vi "sweep init checklist.vi"(9 "list":string[](array[string])=["tabs: init", "gas flow: init", "PID: init", "save log: init", "overheat: init", "counter: init", "sweep table: init", "9ctl: init"], 10 "init str":string, 11 "action":string="action") -> (3 "result":bool)   [LabVIEW 2015]
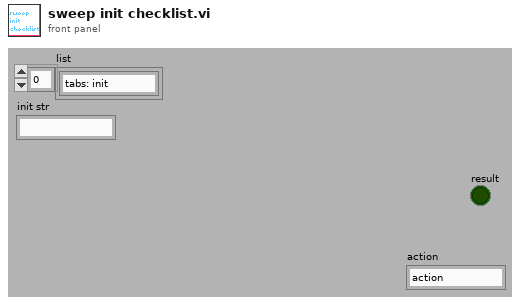
[diagram p1: front panel]
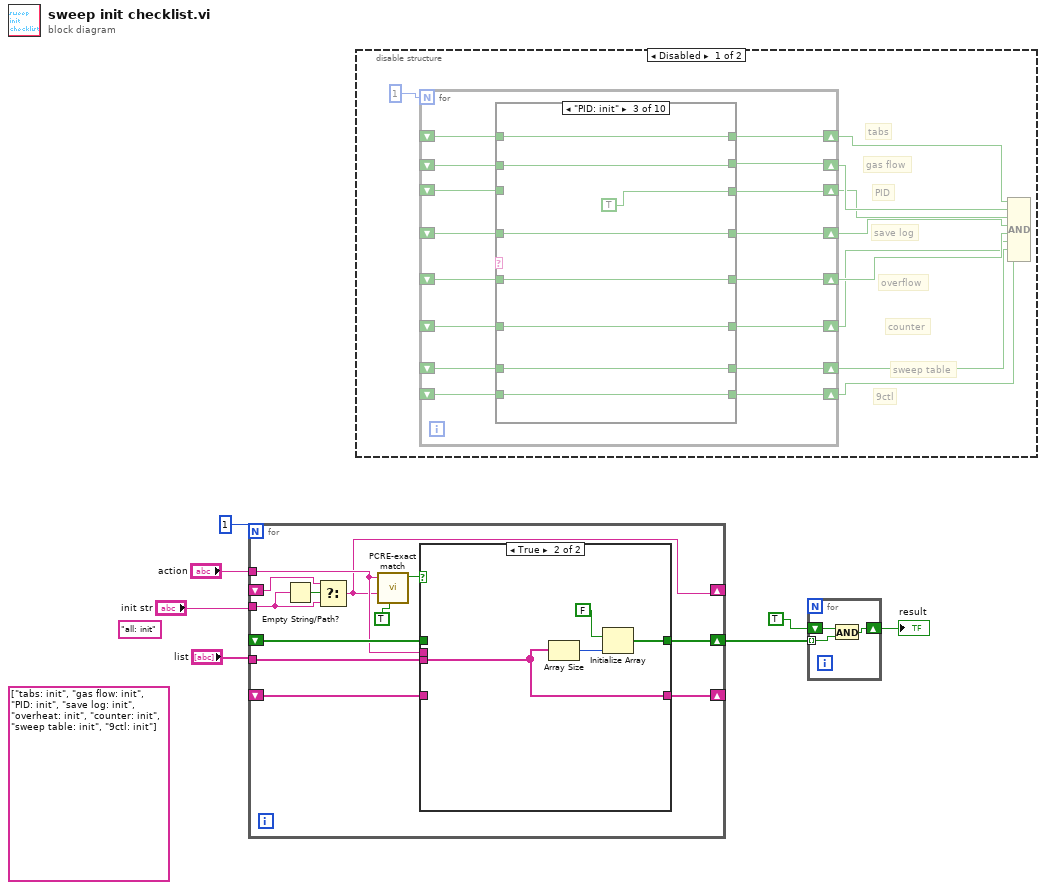
[diagram p0: block diagram]
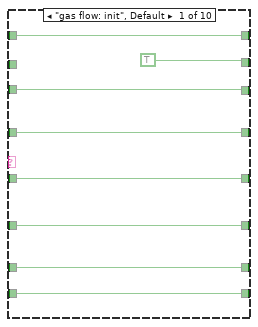
[diagram p2: hidden frame]
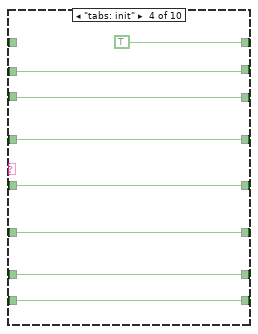
[diagram p4: hidden frame]
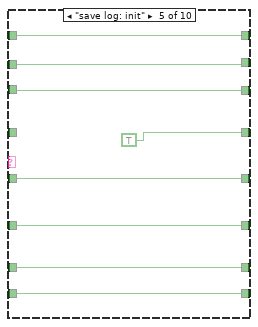
[diagram p5: hidden frame]
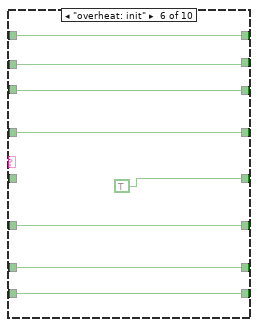
[diagram p6: hidden frame]
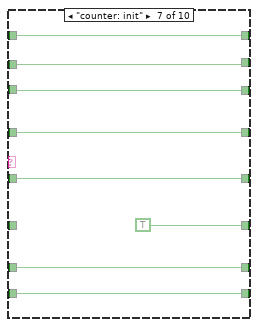
[diagram p7: hidden frame]
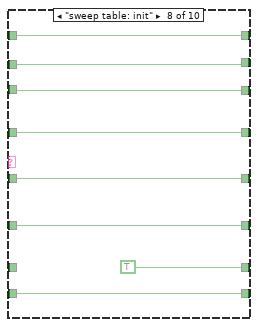
[diagram p8: hidden frame]
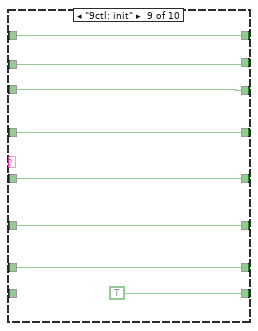
[diagram p9: hidden frame]
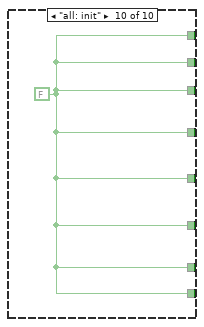
[diagram p10: hidden frame]
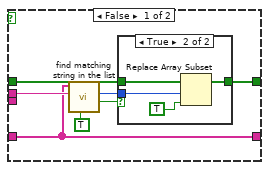
[diagram p12: hidden frame]
diagram:
  (unwired) "all: init" ("regular expression")
  (unwired) string[] ["tabs: init", "gas flow: init", "PID: init", "save log: init", "overheat: init", "counter: init", "sweep table: init", "9ctl: init"]
  n1 = for {
    N: 1 -> [_]
    tunnel: "action" -> [w12]
    shift-right: [w14] -> w5
    shift-left: _ -> [w17]
    shift-right: [w13] -> _
    shift-left: _ -> [w15]
    tunnel: "list" -> [w16]
    tunnel: "init str" -> [w9]
    shift-right: [w8] -> _
    shift-left: _ -> [w10]
    n2 = Empty String/Path?(string/path=w9) -> (empty?=w11:bool)
    n3 = Select(t=w10, s=w11, f=w9) -> (s? t:f=w8:string)
    n4 = call "PCRE-exact match.vi"("quote specials"=TRUE, "regular expression"=w8, "input string"=w12) -> ("exact match"=w18:bool)  [unwired: 6 in, 2 out]
    n5 = case shown="True" w18 {
      tunnel: [w20 w35] -> w14
      tunnel: w17 -> [w22 _]
      tunnel: [w21 w32] -> w13
      tunnel: w16 -> [_ w32]
      tunnel: w15 -> [w21 _]
      tunnel: w12 -> [w23 _]
      frame False {
        n6 = call "find matching string in the list.vi"("quote specials"=TRUE, "regular expression"=w23, "strings"=w21) -> ("match found"=w25:bool, "matching string index"=w26:i32)  [unwired: 6 in, 1 out]
        n7 = case shown="True" w25 {
          tunnel: w26 -> [_ w30]
          tunnel: [w27 w29] -> w20
          tunnel: w22 -> [w27 w28]
          frame False {
          }
          frame True {
            n8 = Replace Array Subset(array=w28, new element=TRUE, index=w30) -> (w29:bool[])
          }
        }
      }
      frame True {
        n9 = Array Size(array=w32) -> (size(s)=w33:i32)
        n10 = Initialize Array(FALSE, w33) -> (w35:bool[])
      }
    }
  }
  n11 = disable-structure shown="Disabled" {
    frame Disabled {
      # "9ctl"
      # "tabs"
      # "sweep table"
      # "counter"
      # "overflow"
      # "save log"
      # "PID"
      # "gas flow"
      n12 = for {
        N: 1 -> [_]
        shift-right: [w60] -> w43
        shift-left: _ -> [w49]
        shift-right: [w59] -> w42
        shift-left: _ -> [w54]
        shift-right: [w58] -> w41
        shift-left: _ -> [w53]
        shift-right: [w57] -> w40
        shift-left: _ -> [w52]
        shift-right: [w56] -> w39
        shift-left: _ -> [w51]
        shift-right: [w55] -> w38
        shift-left: _ -> [w50]
        shift-right: [w48] -> w37
        shift-left: _ -> [w47]
        shift-right: [w46] -> w36
        shift-left: _ -> [w45]
        n13 = case shown="\"PID: init\"" {
          selector: _ -> [_ _ _ _ _ _ _ _ _ _]
          tunnel: [TRUE w70 w80 w88 w97 w106 w115 w124 w131 w133] -> w60
          tunnel: [w67 w76 TRUE w87 w96 w105 w114 w123 w130 w133] -> w59
          tunnel: [w66 w75 w84 w92 TRUE w104 w113 w122 w129 w133] -> w58
          tunnel: [w65 w74 w83 w91 w100 TRUE w112 w121 w128 w133] -> w57
          tunnel: [w64 w73 w82 w90 w99 w108 TRUE w120 w127 w133] -> w56
          tunnel: [w63 w72 w81 w89 w98 w107 w116 TRUE w126 w133] -> w55
          tunnel: w54 -> [w67 w76 _ w87 w96 w105 w114 w123 w130 _]
          tunnel: w53 -> [w66 w75 w84 w92 _ w104 w113 w122 w129 _]
          tunnel: w52 -> [w65 w74 w83 w91 w100 _ w112 w121 w128 _]
          tunnel: w51 -> [w64 w73 w82 w90 w99 w108 _ w120 w127 _]
          tunnel: w50 -> [w63 w72 w81 w89 w98 w107 w116 _ w126 _]
          tunnel: w49 -> [_ w70 w80 w88 w97 w106 w115 w124 w131 _]
          tunnel: [w62 w71 w78 TRUE w94 w102 w110 w118 w132 w133] -> w48
          tunnel: w47 -> [w62 w71 w78 _ w94 w102 w110 w118 w132 _]
          tunnel: [w61 w69 w77 w85 w93 w101 w109 w117 TRUE w133] -> w46
          tunnel: w45 -> [w61 w69 w77 w85 w93 w101 w109 w117 _ _]
          frame "gas flow: init", Default {
          }
          frame "test" {
          }
          frame "PID: init" {
          }
          frame "tabs: init" {
          }
          frame "save log: init" {
          }
          frame "overheat: init" {
          }
          frame "counter: init" {
          }
          frame "sweep table: init" {
          }
          frame "9ctl: init" {
          }
          frame "all: init" {
            w133 = FALSE
          }
        }
      }
      n14 = Compound Arithmetic op=AND(w37, w43, w42, w41, w40, w39, w38, w36) -> ()  [unwired: 1 out]
    }
    frame Enabled {
    }
  }
  n15 = for {
    tunnel: w5 -> [w134] mode=indexing
    shift-right: [w135] -> w3
    shift-left: TRUE -> [w136]
    n16 = And(x=w136, y=w134) -> (x .and. y?=w135:bool)
  }
  "result" <- w3
